vi "读取接收事件引用.vi"(8 "error in (no error)":errorcluster caption="错误输入（无错误）", 11 "上位机 输入":refnum<class "上位机.lvclass">) -> (0 "error out":errorcluster caption="错误输出", 2 "接收数据用户事件":refnum<user-event>, 3 "上位机 输出":refnum<class "上位机.lvclass">)   [LabVIEW 2015, in "上位机.lvlib" / "上位机.lvclass"]
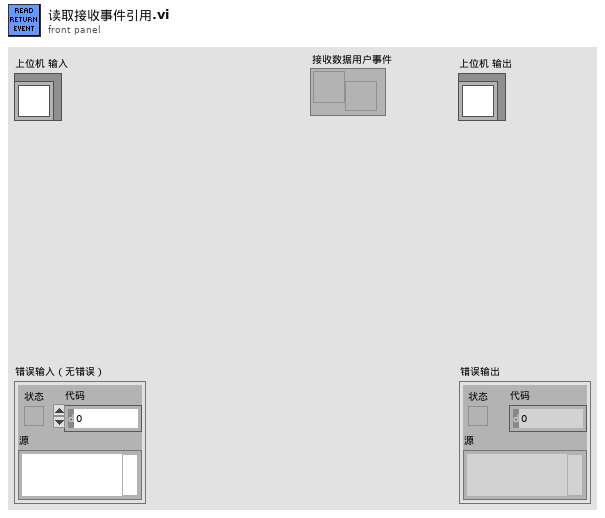
[diagram p1: front panel]
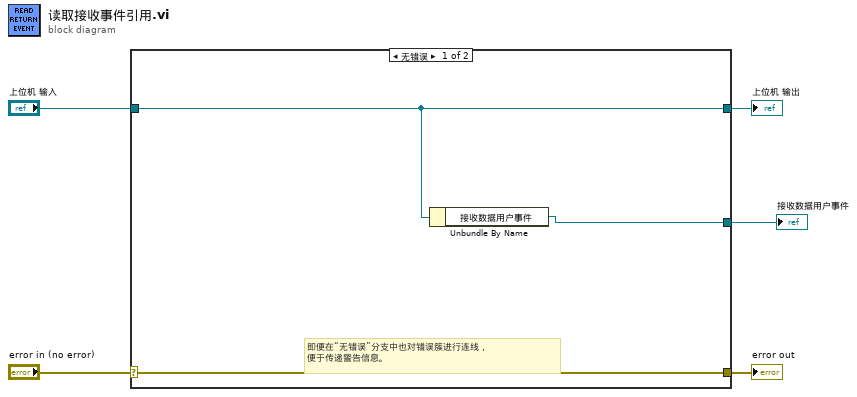
[diagram p0: block diagram]
diagram:
  n1 = case shown="无错误" "error in (no error)" {
    selector: "error in (no error)" -> [w8 w10]
    tunnel: [w8 w10] -> w4
    tunnel: [w7 w9] -> w2
    tunnel: "上位机 输入" -> [w7 w9]
    tunnel: [w6 _] -> w1
    frame No Error {
      # "即便在“无错误”分支中也对错误簇进行连线，\n便于传递警告信息。"
      n2 = Unbundle By Name(w7) -> ("接收数据用户事件"=w6:refnum<user-event>)
    }
    frame Error {
    }
  }
  "error out" <- w4
  "上位机 输出" <- w2
  "接收数据用户事件" <- w1
